vi "Z900_navX_Internal_Get.vi"(8 "error in (no error)":errorcluster, 11 "navX Device":T1={"Interface"={"Protocol"=enum."SERIAL", "Update Rate (4Hz-100Hz)"=4, "navX Open TypeDef"=variant}, "Notify Packet"=refnum, "Loop VI Refnum"=refnum, "Ready to Close Occurrence Refnum"=refnum} {"Interface"."Update Rate (4Hz-100Hz)" min=4 max=60 step=1}) -> (0 "error out":errorcluster, 1 "Connected":bool, 2 "Registry":u8[](array[numeric]), 3 "navX Device":T1={"Interface"={"Protocol"=enum."SERIAL", "Update Rate (4Hz-100Hz)"=4, "navX Open TypeDef"=variant}, "Notify Packet"=refnum, "Loop VI Refnum"=refnum, "Ready to Close Occurrence Refnum"=refnum} {"Interface"."Update Rate (4Hz-100Hz)" min=4 max=60 step=1})   [LabVIEW 2015, in "navX Library v2.lvlib"]
doc: "This VI returns the current values from the navX device registy. This VI is rarely need to be called by a user."
uses:
  navX Library v2.lvlib
  _TypeDefs/Z900_navX_DeviceTypeDef.ctl
  _TypeDefs/Z900_navX_ProtocolTypeDef.ctl
  _TypeDefs/Z900_navX_NotifyPacketTypeDef.ctl
  _TypeDefs/Z900_navX_ActionTypeDef.ctl
  _TypeDefs/Z900_navX_DeviceProcessingLoopStatus.ctl
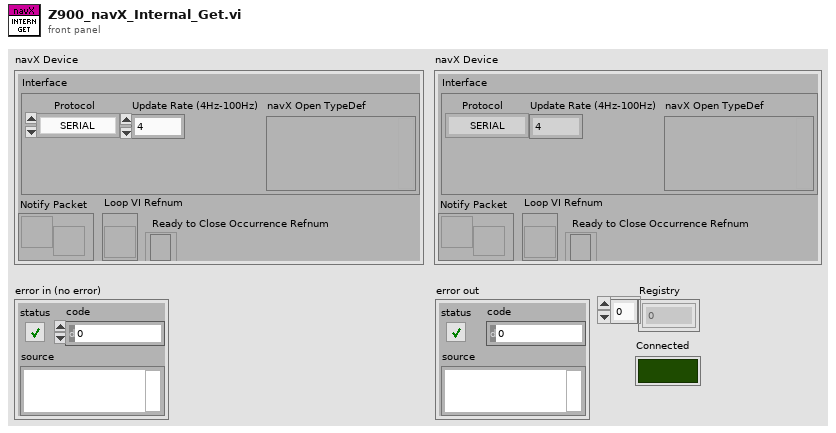
[diagram p1: front panel]
types:
  T1 = typedef "navX Library v2.lvlib/Z900_navX_DeviceTypeDef.ctl" = cluster{"Interface":cluster{"Protocol":T2, "Update Rate (4Hz-100Hz)":u8, "navX Open TypeDef":variant}, "Notify Packet":refnum<notifier>, "Loop VI Refnum":refnum<vi>, "Ready to Close Occurrence Refnum":refnum<k4>}
  T2 = typedef "navX Library v2.lvlib/Z900_navX_ProtocolTypeDef.ctl" = enum16{"SERIAL", "I2C", "SPI"}
  T3 = typedef "navX Library v2.lvlib/Z900_navX_DeviceProcessingLoopStatus.ctl" = cluster{"Registry":u8[], "Connected":bool}
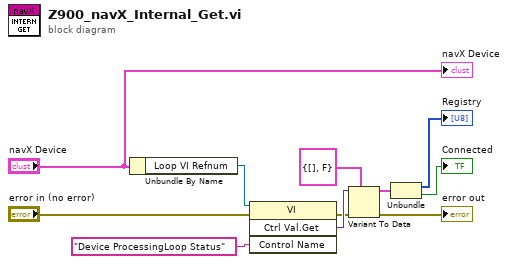
[diagram p0: block diagram]
diagram:
  n1 = Unbundle By Name("navX Device") -> ("Loop VI Refnum"=w9:refnum<vi>)
  n2 = invoke class="VI" method="Ctrl Val.Get"(reference=w9, error in="error in (no error)", "Control Name"="Device ProcessingLoop Status") -> (error out=w5:errorcluster, "Get Control Value Variant"=w6:variant)  [unwired: 1 in, 2 out]
  n3 = Variant To Data(error in=w5, type=T3 {"Registry"=[], "Connected"=FALSE} ("Device ProcessingLoop Status"), Variant=w6) -> (data=w3:T3, error out=→"error out":errorcluster)
  n4 = Unbundle(w3) -> ("Registry"=→"Registry":u8[], "Connected"=→"Connected":bool)
  "navX Device" <- "navX Device"
